vi "hcam_chart_init.vi"() -> ()   [LabVIEW 2020]
uses:
  Typedefs/hcam_data_state.ctl
panel:
  out "state in":T1
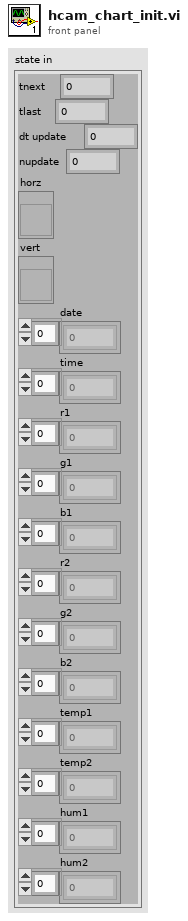
[diagram p1: front panel]
types:
  T1 = typedef "hcam_data_state.ctl" = cluster{"tnext":dbl, "tlast":dbl, "dt update":dbl, "nupdate":i32, "horz":refnum<vi>, "vert":refnum<vi>, "date":dbl[], "time":dbl[], "r1":dbl[], "g1":dbl[], "b1":dbl[], "r2":dbl[], "g2":dbl[], "b2":dbl[], "temp1":dbl[], "temp2":dbl[], "hum1":dbl[], "hum2":dbl[]}
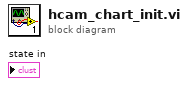
[diagram p0: block diagram]
diagram:
